vi "IV-Trace_v1.1.vi"() -> ()   [LabVIEW 2014]
doc: "This example shows how to configure a measurement and take a reading."
uses:
  <vilib>/Analysis/baseanly.llb/Mean (DBL).vi
  <instrlib>/Keithley 24XX/Public/Data/Read (Single Point).vi
  <vilib>/MakerHub/LINX/Public/Peripherals/Analog/Analog Read 1 Chan.vi
  <instrlib>/Keithley 24XX/Keithley 24XX.lvlib
  <instrlib>/Tektronix TDS 200 1000 2000 Series/Tektronix TDS 200 1000 2000 Series.lvlib
  <vilib>/Analysis/NI_AALBase.lvlib
  <vilib>/MakerHub/LINX/LMH-LINX.lvlib
panel:
  in  "AI Channel":u8
  in  "Serial Port":refnum<visa-resource-name>
  out "Loop Rate (Hz)":u32
  out "Data A0-CH1":string
  in  "File Path Oscillscope":path=path "c:/myfile.txt"
  out "A0 Arduino-CH1 Osc":cluster{"Y":dbl[], dbl[]}(graph)
  in  "Oscilloscope CH1 Probe Attenuation (0.1)":dbl=10.0
  in  "Oscilloscope Source (0: Channel 1)":u16(ring) items=["Channel 1", "Channel 2", "Channel 3", "Channel 4", "Math", "Reference A", "Reference B", "Reference C", "Reference D"]
  in  "Serial Configuration Oscilloscope":T1={"Baud Rate"=9600, "Parity"=0, "Stop Bits"=10, "Flow Control"=2} {"Flow Control" items=["None", "XON/XOFF", "RTS/CTS", "XON/XOFF & RTS/CTS", "DTR/DSR", "XON/XOFF & DTR/DSR"]; "Stop Bits" items=["1.0"=10, "1.5"=15, "2.0"=20]; "Parity" items=["None", "Odd", "Even", "Mark", "Space"]; "Baud Rate" items=["300"=300, "600"=600, "1200"=1200, "2400"=2400, "4800"=4800, "9600"=9600, "19200"=19200]}
  in  "Oscilloscope CH1 Timeout (10000 ms)":u32=10000
  in  "Oscilloscope VISA":refnum<visa-resource-name>
  in  "current multiplier":dbl
  out "Resistance-Time":sgl[](graph)
  out "spreadsheet string":string
  in  "File Path":path=path "c:/myfile.txt"
  out "IV Curve":cluster{sgl[], dbl[]}(graph)
  in  "Stop Voltage/Current":dbl
  in  "Step":dbl
  in  "Source Mode  (0: Voltage)":u16(ring) items=["Voltage", "Current"]
  in  "Compliance  Level (0.1)":dbl=0.1
  in  "Start Voltage/Current":dbl
  in  "Enable Resistance Auto Range (T:Enable)":bool=TRUE
  in  "Enable Current Auto Range (T:Enable)":bool=TRUE
  in  "Enable Voltage Auto Range (T:Enable)":bool=TRUE
  in  "Resistance Manual Range (1.0)":dbl=1.0
  in  "Current Manual Range (1.0)":dbl=1.0
  in  "Voltage Manual Range (1.0)":dbl=1.0
  out "Resistance":sgl
  out "Current":sgl
  out "Voltage":sgl
  in  "Serial Configuration Keithley":T2={"Baud Rate"=9600, "Parity"=0, "Data Bits"=8, "Stop Bits"=10, "Flow Control"=0} {"Flow Control" items=["None", "XON/XOFF", "RTS/CTS", "XON/XOFF & RTS/CTS", "DTR/DSR", "XON/XOFF & DTR/DSR"]; "Stop Bits" items=["1.0"=10, "1.5"=15, "2.0"=20]; "Data Bits" items=["7"=7, "8"=8]; "Parity" items=["None", "Odd", "Even", "Mark", "Space"]; "Baud Rate" items=["300"=300, "600"=600, "1200"=1200, "2400"=2400, "4800"=4800, "9600"=9600, "19200"=19200]}
  in  "VISA resource name":refnum<visa-resource-name>
  # "NanoBEEs 2015-IV Tracer v1.0"
  # "Source Settings"
  # "GPIB9::24::INSTR"
  # "Voltage Range Settings"
  # "Current Range Settings"
  # "This multiplies the current value\nwith the number that entered, in order\nto  graph lower current values."
  # "Resistance Range Settings"
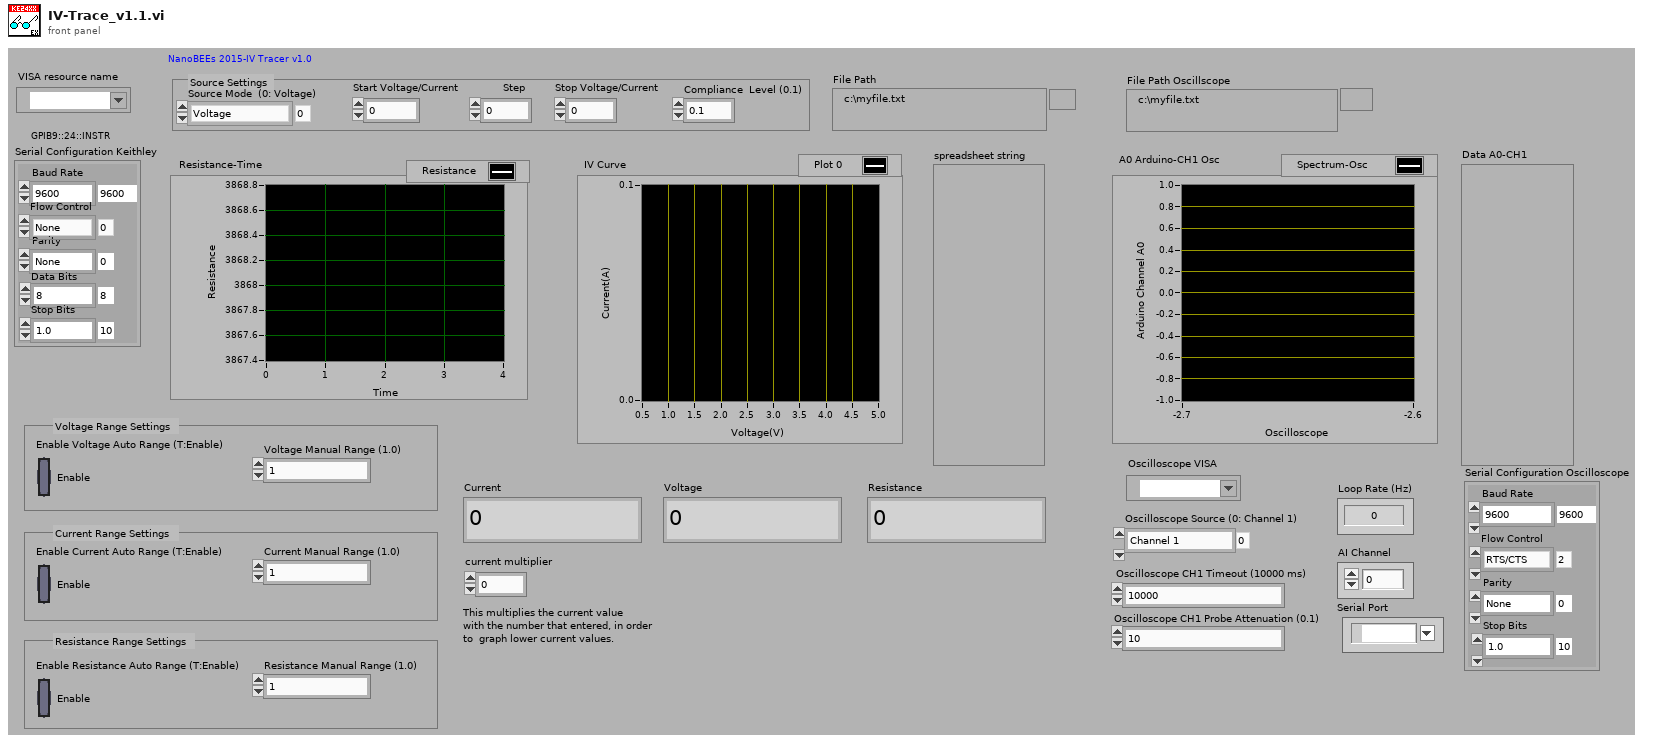
[diagram p1: front panel]
types:
  T1 = cluster{"Baud Rate":u32, "Parity":u16, "Stop Bits":u16, "Flow Control":u16}
  T2 = cluster{"Baud Rate":u32, "Parity":u16, "Data Bits":u16, "Stop Bits":u16, "Flow Control":u16}
  T3 = enum16{"open", "replace", "create", "open or create", "replace or create", "replace or create with confirmation"}
  T4 = typedef "LMH-LINX.lvlib/LINX Ref.ctl" = cluster{"Platform":T5, "Interface":T6, "LINX Device Config":T7}
  T5 = typedef "LMH-LINX.lvlib/Platform.ctl" = enum16{"LINX", "myRIO"}
  T6 = typedef "LMH-LINX.lvlib/Interface.ctl" = enum16{"Serial", "TCP"}
  T7 = typedef "LMH-LINX.lvlib/Device.lvlib/LINX Device Config.ctl" = cluster{"Interface":T6, "COM Port":refnum<visa-resource-name>, "TCP Configuration":T8, "Device Family":u8, "Device ID":u8, "Device Name":string, "TCP Ref":refnum<k5>, "Channels":T9}
  T8 = typedef "LMH-LINX.lvlib/Device.lvlib/TCP Config.ctl" = cluster{"IP Address":string, "Port":u16}
  T9 = typedef "LMH-LINX.lvlib/Channels.ctl" = cluster{"DI":u8[], "DO":u8[], "AI":u8[], "AO":u8[], "PWM":u8[], "QE":u8[], "UART":u8[], "I2C 2":u8[], "SPI":u8[], "CAN":u8[], "Servo":u8[], "AI Ref (V)":dbl, "AO Ref (V)":dbl, "AO Resolution (Bits)":u8}
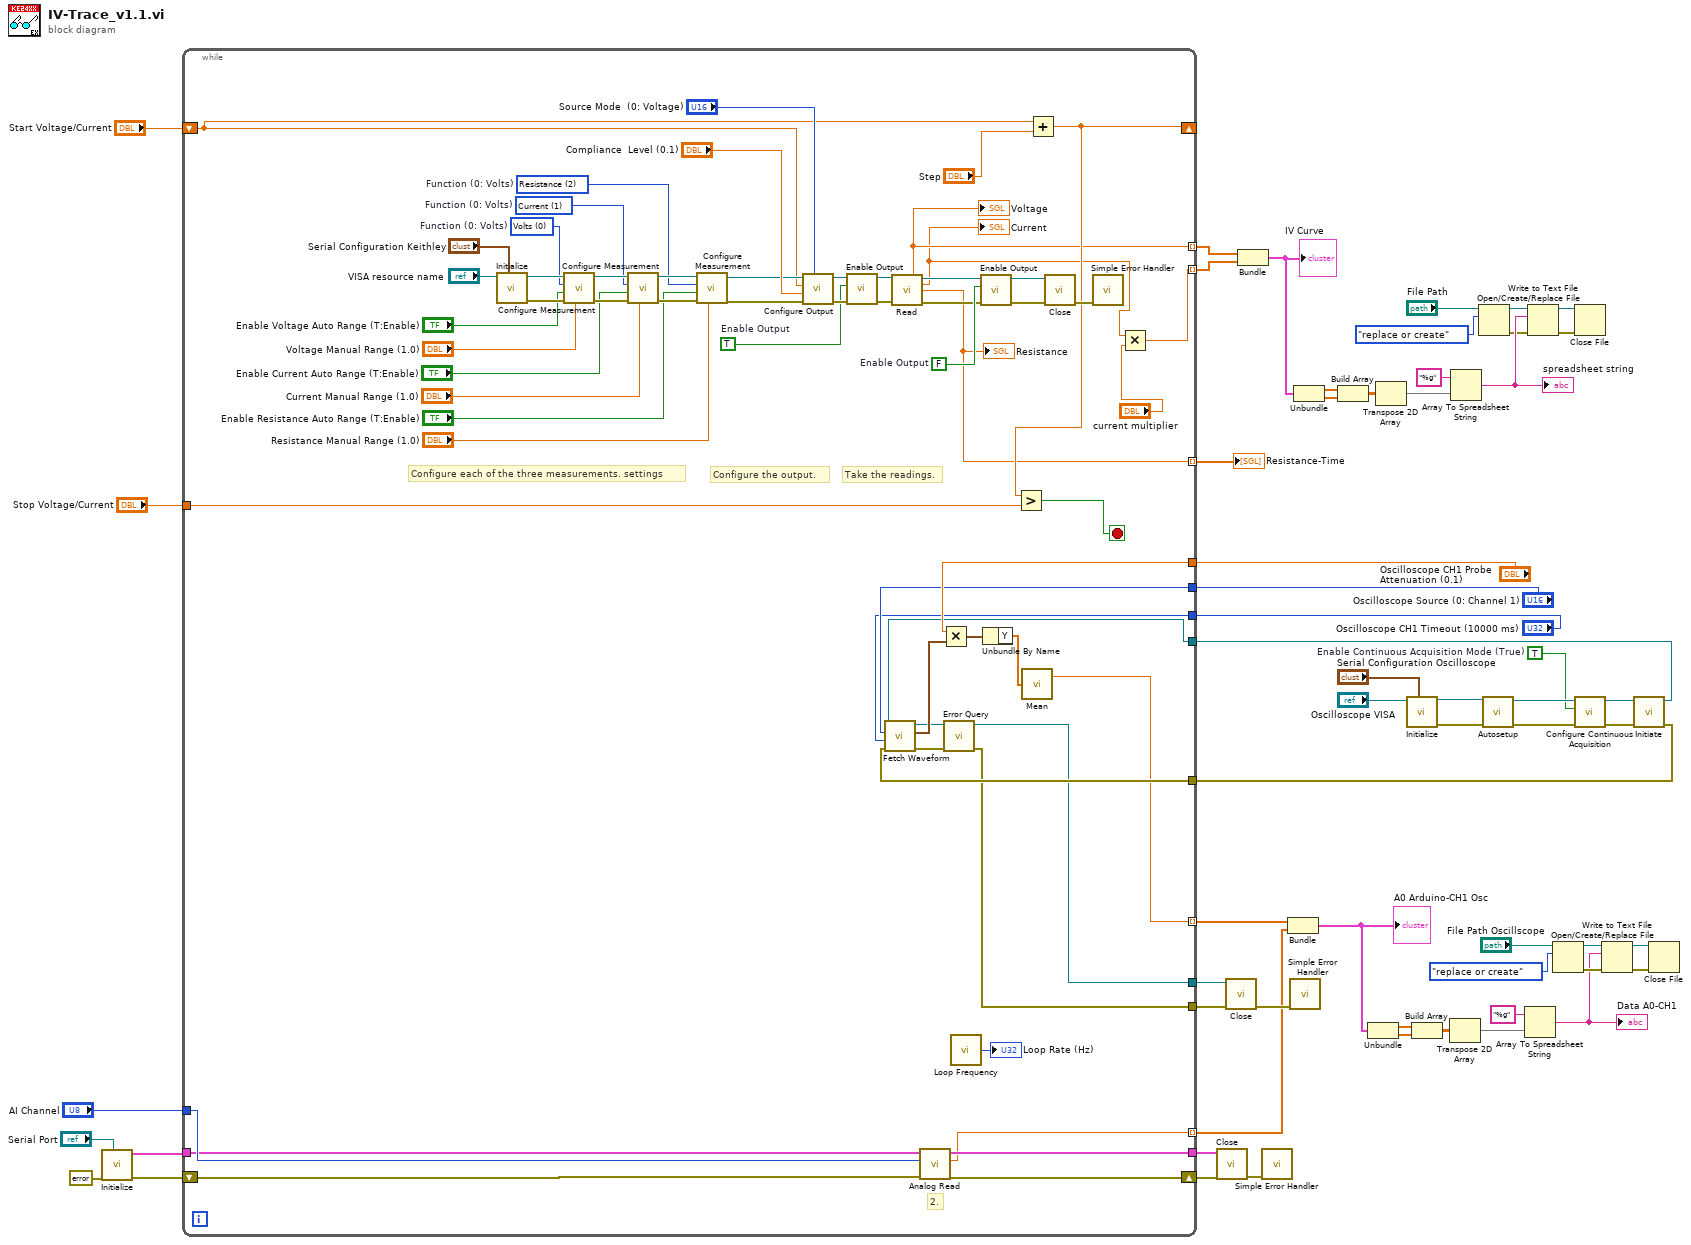
[diagram p0: block diagram]
diagram:
  w34 = TRUE  # Enable Continuous Acquisition Mode (True)
  n1 = call <instrlib>:"Initialize.vi"("Serial Port"="Serial Port", "Error In"=errorcluster {"status"=FALSE, "code"=0, "source"=""}) -> ("Error Out"=w4:errorcluster, "LINX Ref"=w5:T4)  [unwired: 7 in, 1 out]
  n2 = call <instrlib>:"Initialize.vi"("Serial Configuration"="Serial Configuration Oscilloscope", "VISA resource name"="Oscilloscope VISA") -> ("error out"=w39:errorcluster, "VISA resource name out"=w38:refnum<visa-resource-name>)  [unwired: 3 in, 5 out]
  n3 = Open/Create/Replace File(file path (use dialog)="File Path", operation (0:open)=T3."replace or create") -> (refnum out=w49:refnum<file>, error out=w44:errorcluster)  [unwired: 4 in, 1 out]
  n4 = call <instrlib>:"Autosetup.vi"("error in (no error)"=w39, "VISA resource name"=w38) -> ("error out"=w36:errorcluster, "VISA resource name out"=w35:refnum<visa-resource-name>)  [unwired: 8 out]
  n5 = Open/Create/Replace File(file path (use dialog)="File Path Oscillscope", operation (0:open)=T3."replace or create") -> (refnum out=w20:refnum<file>, error out=w25:errorcluster)  [unwired: 4 in, 1 out]
  n6 = call <instrlib>:"Configure Continuous Acquisition.vi"("error in (no error)"=w36, "Enable Continuous Acquisition Mode (True)"=w34, "VISA resource name"=w35) -> ("error out"=w33:errorcluster, "VISA resource name out"=w32:refnum<visa-resource-name>)  [unwired: 7 out]
  n7 = call <instrlib>:"Initiate.vi"("error in (no error)"=w33, "VISA resource name"=w32) -> ("error out"=w27:errorcluster, "VISA resource name out"=w28:refnum<visa-resource-name>)  [unwired: 8 out]
  n8 = while {
    shift-right: [w85] -> _
    shift-left: "Start Voltage/Current" -> [w87]
    tunnel: "Stop Voltage/Current" -> [w84]
    tunnel: [w80] -> w43 mode=indexing
    tunnel: [w83] -> w42 mode=indexing
    tunnel: [w82] -> w41 mode=indexing
    tunnel: "Oscilloscope CH1 Probe Attenuation (0.1)" -> [w73]
    tunnel: "Oscilloscope Source (0: Channel 1)" -> [w72]
    tunnel: "Oscilloscope CH1 Timeout (10000 ms)" -> [w71]
    tunnel: w28 -> [w70]
    tunnel: w27 -> [w69]
    tunnel: [w68] -> w12
    tunnel: [w67] -> w11
    tunnel: [w66] -> w10 mode=indexing
    tunnel: "AI Channel" -> [w64]
    tunnel: w5 -> [w63]
    tunnel: [w61] -> w3
    tunnel: [w60] -> w2 mode=indexing
    shift-right: [w59] -> w1
    shift-left: w4 -> [w62]
    stop <- w88 stop-if-true
    w92 = TRUE  # Enable Output
    w102 = FALSE  # Enable Output
    w109 = u16 2 items=["Volts", "Current", "Resistance"]  # Function (0: Volts)
    w110 = u16 1 items=["Volts", "Current", "Resistance"]  # Function (0: Volts)
    w111 = u16 0 items=["Volts", "Current", "Resistance"]  # Function (0: Volts)
    # "2."
    # "Take the readings."
    # "Configure the output."
    # "Configure each of the three measurements. settings"
    n9 = call <instrlib>:"Initialize.vi"("Serial Configuration"="Serial Configuration Keithley", "VISA resource name"="VISA resource name") -> ("error out"=w116:errorcluster, "VISA resource name out"=w117:refnum<visa-resource-name>)  [unwired: 8 in]
    n10 = call <instrlib>:"Configure Measurement.vi"("Manual Range (1.0)"="Voltage Manual Range (1.0)", "error in (no error)"=w116, "Enable Auto Range (T:Enable)"="Enable Voltage Auto Range (T:Enable)", "Function (0: Volts)"=w111, "VISA resource name"=w117) -> ("error out"=w114:errorcluster, "VISA resource name out"=w115:refnum<visa-resource-name>)  [unwired: 5 in]
    n11 = call <instrlib>:"Configure Measurement.vi"("Manual Range (1.0)"="Current Manual Range (1.0)", "error in (no error)"=w114, "Enable Auto Range (T:Enable)"="Enable Current Auto Range (T:Enable)", "Function (0: Volts)"=w110, "VISA resource name"=w115) -> ("error out"=w113:errorcluster, "VISA resource name out"=w112:refnum<visa-resource-name>)  [unwired: 5 in]
    n12 = call <instrlib>:"Configure Measurement.vi"("Manual Range (1.0)"="Resistance Manual Range (1.0)", "error in (no error)"=w113, "Enable Auto Range (T:Enable)"="Enable Resistance Auto Range (T:Enable)", "Function (0: Volts)"=w109, "VISA resource name"=w112) -> ("error out"=w91:errorcluster, "VISA resource name out"=w90:refnum<visa-resource-name>)  [unwired: 5 in]
    n13 = call <instrlib>:"Configure Output.vi"("Source Mode  (0: Voltage)"="Source Mode  (0: Voltage)", "error in (no error)"=w91, "Compliance  Level (0.1)"="Compliance  Level (0.1)", "Output Level (0)"=w87, "VISA resource name"=w90) -> ("error out"=w93:errorcluster, "VISA resource name out"=w94:refnum<visa-resource-name>)  [unwired: 5 in]
    n14 = call <instrlib>:"Enable Output.vi"("error in (no error)"=w93, "Enable Output (T: Enable)"=w92, "VISA resource name"=w94) -> ("error out"=w96:errorcluster, "VISA resource name out"=w95:refnum<visa-resource-name>)  [unwired: 7 in]
    n15 = call <instrlib>:"Fetch Waveform.vi"("error in (no error)"=w69, "Timeout (10000 ms)"=w71, "Source (0: Channel 1)"=w72, "VISA resource name"=w70) -> ("error out"=w75:errorcluster, "Waveform Data"=w77:waveform(dbl), "VISA resource name out"=w74:refnum<visa-resource-name>)  [unwired: 5 out]
    n16 = call-poly <instrlib>:"Read.vi"("VISA resource name"=w95, "error in (no error)"=w96) -> ("Voltage"=w83:sgl, "VISA resource name out"=w97:refnum<visa-resource-name>, "Current"=w81:sgl, "Resistance"=w82:sgl, "error out"=w98:errorcluster)  [unwired: 7 in, 2 out]
    "Voltage" <- w83
    "Current" <- w81
    "Resistance" <- w82
    n17 = call-poly <vilib>:"Analog Read.vi"("Error In"=w62, "Analog Channel"=w64, "LINX Resource"=w63) -> ("Error Out"=w59:errorcluster, "AI Value"=w60:dbl, "LINX Resource"=w61:T4)  [unwired: 5 in, 1 out]
    n18 = Multiply(x=w73, y=w77) -> (x*y=w76:waveform(dbl))
    n19 = call <instrlib>:"Error Query.vi"("error in (no error)"=w75, "VISA resource name"=w74) -> ("error out"=w68:errorcluster, "VISA resource name out"=w67:refnum<visa-resource-name>)  [unwired: 8 out]
    n20 = call <vilib>:"Loop Frequency.vi"() -> ("Loop Rate (Hz)"=→"Loop Rate (Hz)":u32)
    n21 = call <instrlib>:"Enable Output.vi"("error in (no error)"=w98, "Enable Output (T: Enable)"=w102, "VISA resource name"=w97) -> ("error out"=w99:errorcluster, "VISA resource name out"=w100:refnum<visa-resource-name>)  [unwired: 7 in]
    n22 = Unbundle By Name(w76) -> ("Y"=w78:dbl[])
    n23 = call-poly <vilib>:"Mean.vi"("X"=w78) -> ("mean"=w66:dbl)  [unwired: 1 out]
    n24 = Add(x=w87, y="Step") -> (x+y=w85:dbl)
    n25 = Greater?(x=w85, y=w84) -> (0:w88:bool)
    n26 = call <instrlib>:"Close.vi"("error in (no error)"=w99, "VISA resource name"=w100) -> ("error out"=w120:errorcluster)  [unwired: 9 in]
    n27 = call <vilib>:"Simple Error Handler.vi"("error in (no error)"=w120) -> ()  [unwired: 4 in, 5 out]
    n28 = Multiply(x=w81, y="current multiplier") -> (x*y=w80:dbl)
  }
  "Resistance-Time" <- w41
  n29 = call <instrlib>:"Close.vi"("Error In"=w1, "LINX Resource"=w3) -> ("Error Out"=w9:errorcluster)  [unwired: 8 in, 1 out]
  n30 = call <instrlib>:"Close.vi"("error in (no error)"=w12, "VISA resource name"=w11) -> ("error out"=w26:errorcluster)  [unwired: 9 out]
  n31 = Bundle(w42, w43) -> (w50:cluster{sgl[], dbl[]})  [unwired: 1 out]
  "IV Curve" <- w50
  n32 = call <vilib>:"Simple Error Handler.vi"("error in (no error)"=w9) -> ()  [unwired: 4 in, 5 out]
  n33 = Bundle(w10, w2) -> (w13:cluster{dbl[], dbl[]})  [unwired: 1 out]
  "A0 Arduino-CH1 Osc" <- w13
  n34 = call <vilib>:"Simple Error Handler.vi"("error in (no error)"=w26) -> ()  [unwired: 1 in, 8 out]
  n35 = Unbundle(w50) -> (w51:sgl[], w52:dbl[])
  n36 = Build Array(w51, w52) -> (w53:dbl[][])
  n37 = Unbundle(w13) -> (w19:dbl[], w18:dbl[])
  n38 = Transpose 2D Array(2D array=w53) -> (transposed array=w55:dbl[][])
  n39 = Build Array(w19, w18) -> (w17:dbl[][])
  n40 = Transpose 2D Array(2D array=w17) -> (transposed array=w15:dbl[][])
  n41 = Array To Spreadsheet String(array=w55, 3:"%g" ("format string")) -> (spreadsheet string=w56:string)  [unwired: 1 in]
  "spreadsheet string" <- w56
  n42 = Array To Spreadsheet String(array=w15, 3:"%g" ("format string")) -> (spreadsheet string=w14:string)  [unwired: 1 in]
  "Data A0-CH1" <- w14
  n43 = Write to Text File(file (use dialog)=w49, text=w56, error in=w44) -> (refnum out=w46:refnum<file>, error out=w45:errorcluster)  [unwired: 2 out]
  n44 = Close File(refnum=w46, error in=w45) -> ()  [unwired: 2 out]
  n45 = Write to Text File(file (use dialog)=w20, text=w14, error in=w25) -> (refnum out=w23:refnum<file>, error out=w24:errorcluster)  [unwired: 2 out]
  n46 = Close File(refnum=w23, error in=w24) -> ()  [unwired: 2 out]
